vi "TCP Client 全双工.vi"() -> ()   [LabVIEW 2015]
uses:
  <vilib>/Analysis/NI_AALBase.lvlib
panel:
  out "send data toserver":dbl[](graph)
  in  "stop":bool
  in  "stop 2":bool
  in  "Waveform":waveform(dbl)
  out "receive data from server":waveform(dbl)(graph)
  in  "远程端口":u16
  in  "address":string
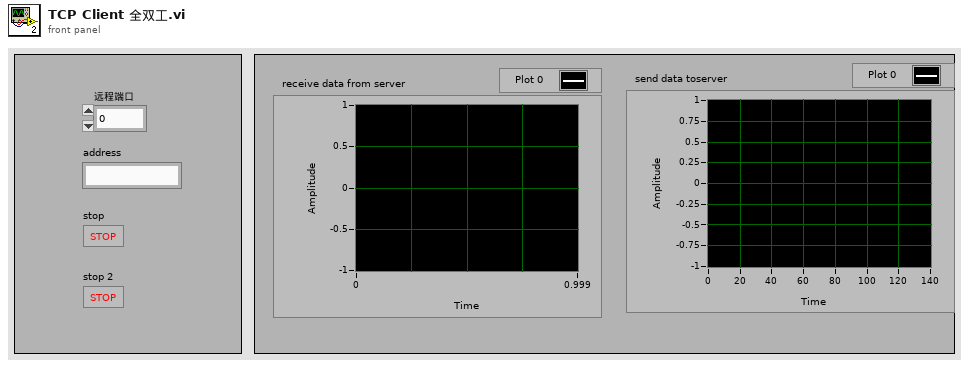
[diagram p1: front panel]
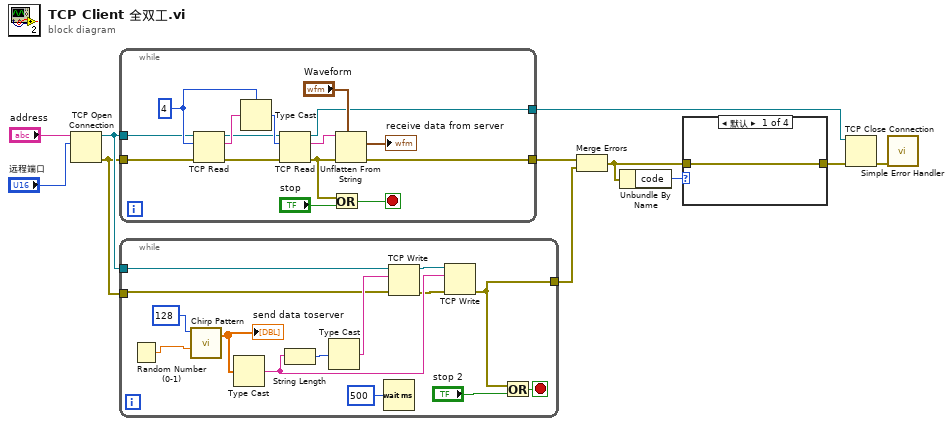
[diagram p0: block diagram]
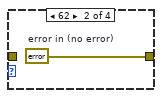
[diagram p2: hidden frame]
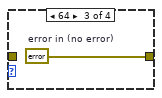
[diagram p3: hidden frame]
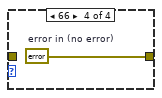
[diagram p4: hidden frame]
diagram:
  n1 = TCP Open Connection(address="address", remote port or service name="远程端口") -> (connection ID=w9:refnum<k5>, error out=w8:errorcluster)  [unwired: 3 in]
  n2 = while {
    tunnel: w8 -> [w20]
    tunnel: w9 -> [w19]
    tunnel: [w16] -> w7
    tunnel: [w15] -> w6
    stop <- w14 stop-if-true
    w24 = 4
    n3 = TCP Read(connection ID=w19, bytes to read=w24, error in (no error)=w20) -> (connection ID out=w22:refnum<k5>, data out=w25:string, error out=w21:errorcluster)  [unwired: 2 in]
    n4 = Type Cast(type=w24, x=w25) -> (*(type *) &x=w26:i32)
    n5 = TCP Read(connection ID=w22, bytes to read=w26, error in (no error)=w21) -> (connection ID out=w16:refnum<k5>, data out=w23:string, error out=w12:errorcluster)  [unwired: 2 in]
    n6 = Or(x=w12, y="stop") -> (x .or. y?=w14:bool)
    n7 = Unflatten From String(type="Waveform", binary string=w23, error in (no error)=w12) -> (value=→"receive data from server":waveform(dbl), error out=w15:errorcluster)  [unwired: 2 in, 1 out]
  }
  n8 = while {
    tunnel: w9 -> [w34]
    tunnel: w8 -> [w33]
    tunnel: [w31] -> w5
    stop <- w30 stop-if-true
    n9 = Random Number (0-1)() -> (number: 0 to 1=w27:dbl)
    n10 = call <vilib>:"Chirp Pattern.vi"("f1"=w27, "samples"=128) -> ("Chirp Pattern"=w29:dbl[])  [unwired: 2 in, 1 out]
    "send data toserver" <- w29
    n11 = Type Cast(x=w29) -> (*(type *) &x=w37:string)  [unwired: 1 in]
    n12 = String Length(string=w37) -> (length=w38:i32)
    n13 = Type Cast(x=w38) -> (*(type *) &x=w39:string)  [unwired: 1 in]
    n14 = Wait (ms)(milliseconds to wait=u32 500) -> ()  [unwired: 1 out]
    n15 = TCP Write(connection ID=w34, data in=w39, error in (no error)=w33) -> (connection ID out=w36:refnum<k5>, error out=w35:errorcluster)  [unwired: 1 in, 1 out]
    n16 = TCP Write(connection ID=w36, data in=w37, error in (no error)=w35) -> (error out=w31:errorcluster)  [unwired: 1 in, 2 out]
    n17 = Or(x=w31, y="stop 2") -> (x .or. y?=w30:bool)
  }
  n18 = Merge Errors(w6, w5) -> (w3:errorcluster)
  n19 = Unbundle By Name(w3) -> ("code"=w4:i32)
  n20 = case shown="默认" w4 {
    tunnel: w3 -> [w41 _ _ _]
    tunnel: [w41 w42 w43 w44] -> w2
    frame Default {
    }
    frame 62 {
      w42 = errorcluster {"status"=TRUE, "code"=0, "source"=""}  # error in (no error)
    }
    frame 64 {
      w43 = errorcluster {"status"=TRUE, "code"=0, "source"=""}  # error in (no error)
    }
    frame 66 {
      w44 = errorcluster {"status"=TRUE, "code"=0, "source"=""}  # error in (no error)
    }
  }
  n21 = TCP Close Connection(connection ID=w7, error in (no error)=w2) -> (error out=w1:errorcluster)  [unwired: 1 in, 1 out]
  n22 = call <vilib>:"Simple Error Handler.vi"("error in (no error)"=w1) -> ()  [unwired: 4 in, 5 out]
